vi "S4GUI.vi"() -> ()   [LabVIEW 2018] (continued)
                n1821 = call-dynamic "save config.vi"("error in (no error)"=w4317, "file config"="lastsaved.cfg", "Channel in"=w4322) -> ("error out"=w4274:errorcluster, "Channel out"=w4279:refnum<class "Channel.lvclass">)  [unwired: 7 in]
                n1822 = local read "Filter2"() -> (w4273:u8)
                n1823 = call-dynamic "Write Filter.vi"("error in (no error)"=w4274, "Filter"=w4273, "Channel in"=w4279) -> ("error out"=w4292:errorcluster, "Channel out"=w4278:refnum<class "Channel.lvclass">)  [unwired: 7 in]
                n1824 = call-dynamic "Read Interface.vi"("error in (no error)"=w4292, "Channel in"=w4278) -> ("error out"=w4289:errorcluster, "Interface.lvclass"=w4288:refnum<class "Interface.lvclass">, "Channel out"=w4277:refnum<class "Channel.lvclass">)  [unwired: 7 in]
                n1825 = call-dynamic "Write Suffix.vi"("error in (no error)"=w4289, "Suffix"=w4272, "Interface in"=w4288) -> ("error out"=w4280:errorcluster, "Interface out"=w4283:refnum<class "Interface.lvclass">)  [unwired: 7 in]
                n1826 = call-dynamic "Write ObsType.vi"("error in (no error)"=w4280, "ObsType"=w4271, "Interface in"=w4283) -> ("error out"=w4281:errorcluster, "Interface out"=w4284:refnum<class "Interface.lvclass">)  [unwired: 7 in]
                n1827 = call-dynamic "Write Object.vi"("error in (no error)"=w4281, "Object"=w4270, "Interface in"=w4284) -> ("error out"=w4282:errorcluster, "Interface out"=w4285:refnum<class "Interface.lvclass">)  [unwired: 7 in]
                n1828 = call-dynamic "Write Comments.vi"("error in (no error)"=w4282, "Comments"=w4269, "Interface in"=w4285) -> ("error out"=w4286:errorcluster, "Interface out"=w4287:refnum<class "Interface.lvclass">)  [unwired: 7 in]
                n1829 = call-dynamic "Write Observer.vi"("error in (no error)"=w4286, "Observer"=w4268, "Interface in"=w4287) -> ("error out"=w4291:errorcluster, "Interface out"=w4290:refnum<class "Interface.lvclass">)  [unwired: 7 in]
                n1830 = call-dynamic "Write Interface.vi"("error in (no error)"=w4291, "Interface.lvclass"=w4290, "Channel in"=w4277) -> ("error out"=w4275:errorcluster, "Channel out"=w4276:refnum<class "Channel.lvclass">)  [unwired: 7 in]
                n1831 = call-dynamic "Read State Machine.vi"("error in (no error)"=w4275, "Device in"=w4276) -> ("error out"=w4314:errorcluster, "State Machine.lvclass"=w4324:refnum<class "State Machine.lvclass">, "Device out"=w4323:refnum<class "Channel.lvclass">)  [unwired: 7 in]
                n1832 = call-dynamic "Write State.vi"("error in (no error)"=w4314, "State"=60, "State Machine in"=w4324) -> ("error out"=w4315:errorcluster, "State Machine out"=w4325:refnum<class "State Machine.lvclass">)  [unwired: 7 in]
                n1833 = call-dynamic "Write State Machine.vi"("error in (no error)"=w4315, "State Machine.lvclass"=w4325, "Device in"=w4323) -> ("error out"=w4327:errorcluster, "Device out"=w4326:refnum<class "Channel.lvclass">)  [unwired: 7 in]
                n1834 = call-dynamic "Write Channel.vi"("error in (no error)"=w4327, "Channel.lvclass"=w4326, "Acquisition in"=w4298) -> ("error out"=w4293:errorcluster, "Acquisition out"=w4294:refnum<class "Acquisition.lvclass">)  [unwired: 7 in]
              }
            }
            n1835 = case shown="True" w4124 {
              tunnel: [w4328 w4385] -> w4135
              tunnel: [w4329 w4384] -> w4136
              tunnel: w4126 -> [w4329 w4356]
              tunnel: w4125 -> [w4328 w4355]
              tunnel: w4108 -> [_ w4334]
              tunnel: w4107 -> [_ w4333]
              tunnel: w4106 -> [_ w4332]
              tunnel: w4105 -> [_ w4331]
              tunnel: w4104 -> [_ w4330]
              frame False {
              }
              frame True {
                # "nome do arquivo .cfg"
                # "seção no arquivo .cfg"
                # "open"
                n1836 = call-dynamic "Read Channel.vi"("error in (no error)"=w4355, "Acquisition in"=w4356) -> ("error out"=w4386:errorcluster, "Channel.lvclass"=w4387:refnum<class "Channel.lvclass">, "Acquisition out"=w4388:refnum<class "Acquisition.lvclass">)  [unwired: 7 in]
                n1837 = call-dynamic "Read Interface.vi"("error in (no error)"=w4386, "Channel in"=w4387) -> ("error out"=w4376:errorcluster, "Interface.lvclass"=w4375:refnum<class "Interface.lvclass">, "Channel out"=w4389:refnum<class "Channel.lvclass">)  [unwired: 7 in]
                n1838 = call-dynamic "Get CCD_Config.vi"("error in (no error)"=w4376, "Interface in"=w4375) -> ("error out"=w4379:errorcluster, "output cluster"=w4380:T24, "Interface out"=w4374:refnum<class "Interface.lvclass">)  [unwired: 7 in]
                n1839 = Bundle By Name(cluster=w4380, "SHUTTER_MODE"=u8 1) -> (w4378:T24)
                n1840 = call-dynamic "Set CCD_Config.vi"("error in (no error)"=w4379, "input cluster"=w4378, "Interface in"=w4374) -> ("error out"=w4381:errorcluster, "Interface out"=w4373:refnum<class "Interface.lvclass">)  [unwired: 7 in]
                n1841 = Flatten To String(anything=w4378, error in (no error)=w4381) -> (data string=w4383:string, error out=w4382:errorcluster)  [unwired: 2 in, 1 out]
                n1842 = call "Write flatted cluster.vi"("error in (no error)"=w4382, "flatted cluster"=w4383, "Interface in"=w4373) -> ("error out"=w4371:errorcluster, "Interface out"=w4372:refnum<class "Interface.lvclass">)  [unwired: 7 in]
                n1843 = call-dynamic "Write Interface.vi"("error in (no error)"=w4371, "Interface.lvclass"=w4372, "Channel in"=w4389) -> ("error out"=w4366:errorcluster, "Channel out"=w4365:refnum<class "Channel.lvclass">)  [unwired: 7 in]
                n1844 = call "Write section_name.vi"("error in (no error)"=w4366, "section_name"="CCD_ACS1", "Channel in"=w4365) -> ("error out"=w4367:errorcluster, "Channel out"=w4362:refnum<class "Channel.lvclass">)  [unwired: 7 in]
                n1845 = call-dynamic "save config.vi"("error in (no error)"=w4367, "file config"="lastsaved.cfg", "Channel in"=w4362) -> ("error out"=w4338:errorcluster, "Channel out"=w4337:refnum<class "Channel.lvclass">)  [unwired: 7 in]
                n1846 = local read "Filter1"() -> (w4339:u8)
                n1847 = call-dynamic "Write Filter.vi"("error in (no error)"=w4338, "Filter"=w4339, "Channel in"=w4337) -> ("error out"=w4354:errorcluster, "Channel out"=w4353:refnum<class "Channel.lvclass">)  [unwired: 7 in]
                n1848 = call-dynamic "Read Interface.vi"("error in (no error)"=w4354, "Channel in"=w4353) -> ("error out"=w4350:errorcluster, "Interface.lvclass"=w4349:refnum<class "Interface.lvclass">, "Channel out"=w4343:refnum<class "Channel.lvclass">)  [unwired: 7 in]
                n1849 = call-dynamic "Write Suffix.vi"("error in (no error)"=w4350, "Suffix"=w4334, "Interface in"=w4349) -> ("error out"=w4340:errorcluster, "Interface out"=w4344:refnum<class "Interface.lvclass">)  [unwired: 7 in]
                n1850 = call-dynamic "Write ObsType.vi"("error in (no error)"=w4340, "ObsType"=w4333, "Interface in"=w4344) -> ("error out"=w4341:errorcluster, "Interface out"=w4345:refnum<class "Interface.lvclass">)  [unwired: 7 in]
                n1851 = call-dynamic "Write Object.vi"("error in (no error)"=w4341, "Object"=w4332, "Interface in"=w4345) -> ("error out"=w4342:errorcluster, "Interface out"=w4346:refnum<class "Interface.lvclass">)  [unwired: 7 in]
                n1852 = call-dynamic "Write Comments.vi"("error in (no error)"=w4342, "Comments"=w4331, "Interface in"=w4346) -> ("error out"=w4347:errorcluster, "Interface out"=w4348:refnum<class "Interface.lvclass">)  [unwired: 7 in]
                n1853 = call-dynamic "Write Observer.vi"("error in (no error)"=w4347, "Observer"=w4330, "Interface in"=w4348) -> ("error out"=w4352:errorcluster, "Interface out"=w4351:refnum<class "Interface.lvclass">)  [unwired: 7 in]
                n1854 = call-dynamic "Write Interface.vi"("error in (no error)"=w4352, "Interface.lvclass"=w4351, "Channel in"=w4343) -> ("error out"=w4335:errorcluster, "Channel out"=w4336:refnum<class "Channel.lvclass">)  [unwired: 7 in]
                n1855 = call-dynamic "Read State Machine.vi"("error in (no error)"=w4335, "Device in"=w4336) -> ("error out"=w4370:errorcluster, "State Machine.lvclass"=w4360:refnum<class "State Machine.lvclass">, "Device out"=w4361:refnum<class "Channel.lvclass">)  [unwired: 7 in]
                n1856 = call-dynamic "Write State.vi"("error in (no error)"=w4370, "State"=60, "State Machine in"=w4360) -> ("error out"=w4369:errorcluster, "State Machine out"=w4359:refnum<class "State Machine.lvclass">)  [unwired: 7 in]
                n1857 = call-dynamic "Write State Machine.vi"("error in (no error)"=w4369, "State Machine.lvclass"=w4359, "Device in"=w4361) -> ("error out"=w4357:errorcluster, "Device out"=w4358:refnum<class "Channel.lvclass">)  [unwired: 7 in]
                n1858 = call-dynamic "Write Channel.vi"("error in (no error)"=w4357, "Channel.lvclass"=w4358, "Acquisition in"=w4388) -> ("error out"=w4385:errorcluster, "Acquisition out"=w4384:refnum<class "Acquisition.lvclass">)  [unwired: 7 in]
              }
            }
            n1859 = case shown="True" w4118 {
              tunnel: w4120 -> [w4205 w4234]
              tunnel: w4119 -> [w4204 w4233]
              tunnel: [w4205 w4232] -> w4132
              tunnel: [w4204 w4231] -> w4131
              tunnel: w4108 -> [_ w4210]
              tunnel: w4107 -> [_ w4209]
              tunnel: w4106 -> [_ w4208]
              tunnel: w4105 -> [_ w4207]
              tunnel: w4104 -> [_ w4206]
              frame False {
              }
              frame True {
                # "nome do arquivo .cfg"
                # "seção no arquivo .cfg"
                # "open"
                n1860 = call-dynamic "Read Channel.vi"("error in (no error)"=w4233, "Acquisition in"=w4234) -> ("error out"=w4238:errorcluster, "Channel.lvclass"=w4237:refnum<class "Channel.lvclass">, "Acquisition out"=w4236:refnum<class "Acquisition.lvclass">)  [unwired: 7 in]
                n1861 = call-dynamic "Read Interface.vi"("error in (no error)"=w4238, "Channel in"=w4237) -> ("error out"=w4246:errorcluster, "Interface.lvclass"=w4247:refnum<class "Interface.lvclass">, "Channel out"=w4235:refnum<class "Channel.lvclass">)  [unwired: 7 in]
                n1862 = call-dynamic "Get CCD_Config.vi"("error in (no error)"=w4246, "Interface in"=w4247) -> ("error out"=w4243:errorcluster, "output cluster"=w4242:T24, "Interface out"=w4248:refnum<class "Interface.lvclass">)  [unwired: 7 in]
                n1863 = Bundle By Name(cluster=w4242, "SHUTTER_MODE"=u8 1) -> (w4244:T24)
                n1864 = call-dynamic "Set CCD_Config.vi"("error in (no error)"=w4243, "input cluster"=w4244, "Interface in"=w4248) -> ("error out"=w4241:errorcluster, "Interface out"=w4249:refnum<class "Interface.lvclass">)  [unwired: 7 in]
                n1865 = Flatten To String(anything=w4244, error in (no error)=w4241) -> (data string=w4239:string, error out=w4240:errorcluster)  [unwired: 2 in, 1 out]
                n1866 = call "Write flatted cluster.vi"("error in (no error)"=w4240, "flatted cluster"=w4239, "Interface in"=w4249) -> ("error out"=w4251:errorcluster, "Interface out"=w4250:refnum<class "Interface.lvclass">)  [unwired: 7 in]
                n1867 = call-dynamic "Write Interface.vi"("error in (no error)"=w4251, "Interface.lvclass"=w4250, "Channel in"=w4235) -> ("error out"=w4256:errorcluster, "Channel out"=w4257:refnum<class "Channel.lvclass">)  [unwired: 7 in]
                n1868 = call "Write section_name.vi"("error in (no error)"=w4256, "section_name"="CCD_ACS3", "Channel in"=w4257) -> ("error out"=w4255:errorcluster, "Channel out"=w4260:refnum<class "Channel.lvclass">)  [unwired: 7 in]
                n1869 = call-dynamic "save config.vi"("error in (no error)"=w4255, "file config"="lastsaved.cfg", "Channel in"=w4260) -> ("error out"=w4212:errorcluster, "Channel out"=w4215:refnum<class "Channel.lvclass">)  [unwired: 7 in]
                n1870 = local read "Filter3"() -> (w4211:u8)
                n1871 = call-dynamic "Write Filter.vi"("error in (no error)"=w4212, "Filter"=w4211, "Channel in"=w4215) -> ("error out"=w4216:errorcluster, "Channel out"=w4229:refnum<class "Channel.lvclass">)  [unwired: 7 in]
                n1872 = call-dynamic "Read Interface.vi"("error in (no error)"=w4216, "Channel in"=w4229) -> ("error out"=w4219:errorcluster, "Interface.lvclass"=w4220:refnum<class "Interface.lvclass">, "Channel out"=w4230:refnum<class "Channel.lvclass">)  [unwired: 7 in]
                n1873 = call-dynamic "Write Suffix.vi"("error in (no error)"=w4219, "Suffix"=w4210, "Interface in"=w4220) -> ("error out"=w4228:errorcluster, "Interface out"=w4225:refnum<class "Interface.lvclass">)  [unwired: 7 in]
                n1874 = call-dynamic "Write ObsType.vi"("error in (no error)"=w4228, "ObsType"=w4209, "Interface in"=w4225) -> ("error out"=w4227:errorcluster, "Interface out"=w4224:refnum<class "Interface.lvclass">)  [unwired: 7 in]
                n1875 = call-dynamic "Write Object.vi"("error in (no error)"=w4227, "Object"=w4208, "Interface in"=w4224) -> ("error out"=w4226:errorcluster, "Interface out"=w4223:refnum<class "Interface.lvclass">)  [unwired: 7 in]
                n1876 = call-dynamic "Write Comments.vi"("error in (no error)"=w4226, "Comments"=w4207, "Interface in"=w4223) -> ("error out"=w4222:errorcluster, "Interface out"=w4221:refnum<class "Interface.lvclass">)  [unwired: 7 in]
                n1877 = call-dynamic "Write Observer.vi"("error in (no error)"=w4222, "Observer"=w4206, "Interface in"=w4221) -> ("error out"=w4217:errorcluster, "Interface out"=w4218:refnum<class "Interface.lvclass">)  [unwired: 7 in]
                n1878 = call-dynamic "Write Interface.vi"("error in (no error)"=w4217, "Interface.lvclass"=w4218, "Channel in"=w4230) -> ("error out"=w4213:errorcluster, "Channel out"=w4214:refnum<class "Channel.lvclass">)  [unwired: 7 in]
                n1879 = call-dynamic "Read State Machine.vi"("error in (no error)"=w4213, "Device in"=w4214) -> ("error out"=w4252:errorcluster, "State Machine.lvclass"=w4262:refnum<class "State Machine.lvclass">, "Device out"=w4261:refnum<class "Channel.lvclass">)  [unwired: 7 in]
                n1880 = call-dynamic "Write State.vi"("error in (no error)"=w4252, "State"=60, "State Machine in"=w4262) -> ("error out"=w4253:errorcluster, "State Machine out"=w4263:refnum<class "State Machine.lvclass">)  [unwired: 7 in]
                n1881 = call-dynamic "Write State Machine.vi"("error in (no error)"=w4253, "State Machine.lvclass"=w4263, "Device in"=w4261) -> ("error out"=w4265:errorcluster, "Device out"=w4264:refnum<class "Channel.lvclass">)  [unwired: 7 in]
                n1882 = call-dynamic "Write Channel.vi"("error in (no error)"=w4265, "Channel.lvclass"=w4264, "Acquisition in"=w4236) -> ("error out"=w4231:errorcluster, "Acquisition out"=w4232:refnum<class "Acquisition.lvclass">)  [unwired: 7 in]
              }
            }
            n1883 = case shown="True" w4115 {
              tunnel: w4117 -> [w4143 w4172]
              tunnel: w4116 -> [w4142 w4171]
              tunnel: [w4143 w4170] -> w4130
              tunnel: [w4142 w4169] -> w4129
              tunnel: w4108 -> [_ w4148]
              tunnel: w4107 -> [_ w4147]
              tunnel: w4106 -> [_ w4146]
              tunnel: w4105 -> [_ w4145]
              tunnel: w4104 -> [_ w4144]
              frame False {
              }
              frame True {
                # "nome do arquivo .cfg"
                # "seção no arquivo .cfg"
                # "open"
                n1884 = call-dynamic "Read Channel.vi"("error in (no error)"=w4171, "Acquisition in"=w4172) -> ("error out"=w4200:errorcluster, "Channel.lvclass"=w4201:refnum<class "Channel.lvclass">, "Acquisition out"=w4202:refnum<class "Acquisition.lvclass">)  [unwired: 7 in]
                n1885 = call-dynamic "Read Interface.vi"("error in (no error)"=w4200, "Channel in"=w4201) -> ("error out"=w4192:errorcluster, "Interface.lvclass"=w4191:refnum<class "Interface.lvclass">, "Channel out"=w4203:refnum<class "Channel.lvclass">)  [unwired: 7 in]
                n1886 = call-dynamic "Get CCD_Config.vi"("error in (no error)"=w4192, "Interface in"=w4191) -> ("error out"=w4195:errorcluster, "output cluster"=w4196:T24, "Interface out"=w4190:refnum<class "Interface.lvclass">)  [unwired: 7 in]
                n1887 = Bundle By Name(cluster=w4196, "SHUTTER_MODE"=u8 1) -> (w4194:T24)
                n1888 = call-dynamic "Set CCD_Config.vi"("error in (no error)"=w4195, "input cluster"=w4194, "Interface in"=w4190) -> ("error out"=w4197:errorcluster, "Interface out"=w4189:refnum<class "Interface.lvclass">)  [unwired: 7 in]
                n1889 = Flatten To String(anything=w4194, error in (no error)=w4197) -> (data string=w4199:string, error out=w4198:errorcluster)  [unwired: 2 in, 1 out]
                n1890 = call "Write flatted cluster.vi"("error in (no error)"=w4198, "flatted cluster"=w4199, "Interface in"=w4189) -> ("error out"=w4187:errorcluster, "Interface out"=w4188:refnum<class "Interface.lvclass">)  [unwired: 7 in]
                n1891 = call-dynamic "Write Interface.vi"("error in (no error)"=w4187, "Interface.lvclass"=w4188, "Channel in"=w4203) -> ("error out"=w4182:errorcluster, "Channel out"=w4181:refnum<class "Channel.lvclass">)  [unwired: 7 in]
                n1892 = call "Write section_name.vi"("error in (no error)"=w4182, "section_name"="CCD_ACS4", "Channel in"=w4181) -> ("error out"=w4183:errorcluster, "Channel out"=w4178:refnum<class "Channel.lvclass">)  [unwired: 7 in]
                n1893 = call-dynamic "save config.vi"("error in (no error)"=w4183, "file config"="lastsaved.cfg", "Channel in"=w4178) -> ("error out"=w4150:errorcluster, "Channel out"=w4155:refnum<class "Channel.lvclass">)  [unwired: 7 in]
                n1894 = local read "Filter4"() -> (w4149:u8)
                n1895 = call-dynamic "Write Filter.vi"("error in (no error)"=w4150, "Filter"=w4149, "Channel in"=w4155) -> ("error out"=w4168:errorcluster, "Channel out"=w4154:refnum<class "Channel.lvclass">)  [unwired: 7 in]
                n1896 = call-dynamic "Read Interface.vi"("error in (no error)"=w4168, "Channel in"=w4154) -> ("error out"=w4165:errorcluster, "Interface.lvclass"=w4164:refnum<class "Interface.lvclass">, "Channel out"=w4153:refnum<class "Channel.lvclass">)  [unwired: 7 in]
                n1897 = call-dynamic "Write Suffix.vi"("error in (no error)"=w4165, "Suffix"=w4148, "Interface in"=w4164) -> ("error out"=w4156:errorcluster, "Interface out"=w4159:refnum<class "Interface.lvclass">)  [unwired: 7 in]
                n1898 = call-dynamic "Write ObsType.vi"("error in (no error)"=w4156, "ObsType"=w4147, "Interface in"=w4159) -> ("error out"=w4157:errorcluster, "Interface out"=w4160:refnum<class "Interface.lvclass">)  [unwired: 7 in]
                n1899 = call-dynamic "Write Object.vi"("error in (no error)"=w4157, "Object"=w4146, "Interface in"=w4160) -> ("error out"=w4158:errorcluster, "Interface out"=w4161:refnum<class "Interface.lvclass">)  [unwired: 7 in]
                n1900 = call-dynamic "Write Comments.vi"("error in (no error)"=w4158, "Comments"=w4145, "Interface in"=w4161) -> ("error out"=w4162:errorcluster, "Interface out"=w4163:refnum<class "Interface.lvclass">)  [unwired: 7 in]
                n1901 = call-dynamic "Write Observer.vi"("error in (no error)"=w4162, "Observer"=w4144, "Interface in"=w4163) -> ("error out"=w4167:errorcluster, "Interface out"=w4166:refnum<class "Interface.lvclass">)  [unwired: 7 in]
                n1902 = call-dynamic "Write Interface.vi"("error in (no error)"=w4167, "Interface.lvclass"=w4166, "Channel in"=w4153) -> ("error out"=w4151:errorcluster, "Channel out"=w4152:refnum<class "Channel.lvclass">)  [unwired: 7 in]
                n1903 = call-dynamic "Read State Machine.vi"("error in (no error)"=w4151, "Device in"=w4152) -> ("error out"=w4186:errorcluster, "State Machine.lvclass"=w4176:refnum<class "State Machine.lvclass">, "Device out"=w4177:refnum<class "Channel.lvclass">)  [unwired: 7 in]
                n1904 = call-dynamic "Write State.vi"("error in (no error)"=w4186, "State"=60, "State Machine in"=w4176) -> ("error out"=w4185:errorcluster, "State Machine out"=w4175:refnum<class "State Machine.lvclass">)  [unwired: 7 in]
                n1905 = call-dynamic "Write State Machine.vi"("error in (no error)"=w4185, "State Machine.lvclass"=w4175, "Device in"=w4177) -> ("error out"=w4173:errorcluster, "Device out"=w4174:refnum<class "Channel.lvclass">)  [unwired: 7 in]
                n1906 = call-dynamic "Write Channel.vi"("error in (no error)"=w4173, "Channel.lvclass"=w4174, "Acquisition in"=w4202) -> ("error out"=w4169:errorcluster, "Acquisition out"=w4170:refnum<class "Acquisition.lvclass">)  [unwired: 7 in]
              }
            }
            n1907 = disable-structure shown="Enabled" {
              frame Disabled {
                # "open"
                n1908 = local read "Input Cluster"() -> (w4139:T5)
                n1909 = Unbundle By Name(w4139) -> ("Parameters"=w4140:T23)
                n1910 = Bundle By Name(cluster=w4140, "Shutter\nMode"=u16 1 ("Shutter\nMode")) -> (w4137:T23)
                n1911 = Bundle By Name(cluster=w4139, "Parameters"=w4137) -> (w4138:T5)
                n1912 = local write "Input Cluster"(w4138) -> ()
              }
              frame Enabled {
              }
            }
          }
        }
        n1913 = call-dynamic "Write AcquisitionA.vi"("error in (no error)"=w3698, "Acquisition.lvclass"=w3699, "S4ACS_GUI in"=w3700) -> ("error out"=w3688:errorcluster, "S4ACS_GUI out"=w3692:refnum<class "S4GUI.lvclass">)  [unwired: 7 in]
        n1914 = call "Write AcquisitionB.vi"("error in (no error)"=w3693, "Acquisition.lvclass"=w3694, "S4ACS_GUI in"=w3692) -> ("error out"=w3687:errorcluster, "S4ACS_GUI out"=w3691:refnum<class "S4GUI.lvclass">)  [unwired: 7 in]
        n1915 = call-dynamic "Write AcquisitionC.vi"("error in (no error)"=w3682, "Acquisition.lvclass"=w3683, "S4ACS_GUI in"=w3691) -> ("error out"=w3686:errorcluster, "S4ACS_GUI out"=w3690:refnum<class "S4GUI.lvclass">)  [unwired: 7 in]
        n1916 = call-dynamic "Write AcquisitionD.vi"("error in (no error)"=w3680, "Acquisition.lvclass"=w3681, "S4ACS_GUI in"=w3690) -> ("error out"=w3685:errorcluster, "S4ACS_GUI out"=w3689:refnum<class "S4GUI.lvclass">)  [unwired: 7 in]
        n1917 = Merge Errors(w3688, w3687, w3686, w3685) -> (w3684:errorcluster)
        n1918 = call "Write cfg file.vi"("error in (no error)"=w3684, "cfg file"="lastsaved.cfg", "S4ACS_GUI in"=w3689) -> ("error out"=w3696:errorcluster, "S4ACS_GUI out"=w3695:refnum<class "S4GUI.lvclass">)  [unwired: 7 in]
      }
      event "Object_sflat", "Object_dark", "Object_zero", "Object_dflat", "Object_focus", "Object_obj": Value Change {
        n1919 = event-data() -> ("NewVal"=w4390:string)  [unwired: 1 in, 5 out]
        n1920 = stacked-sequence {
          seq-local: [w4426 _ _ _] -> [_ w4484 _ _]
          seq-local: [w4425 _ _ _] -> [_ w4483 _ _]
          seq-local: [_ w4482 _ _] -> [_ _ w4527 _]
          seq-local: [_ w4481 _ _] -> [_ _ w4526 _]
          seq-local: [_ _ w4525 _] -> [_ _ _ w4570]
          seq-local: [_ _ w4524 _] -> [_ _ _ w4569]
          tunnel: w4397 -> [w4438 _ _ _]
          tunnel: w4398 -> [w4437 _ _ _]
          tunnel: [_ _ _ w4568] -> w4392
          tunnel: [_ _ _ w4567] -> w4391
          tunnel: w4396 -> [w4424 w4480 w4523 w4566]
          tunnel: w4395 -> [w4423 w4479 w4509 w4552]
          tunnel: w4393 -> [w4422 w4465 w4508 w4551]
          tunnel: w4390 -> [w4421 w4464 w4507 w4550]
          tunnel: w4394 -> [w4420 w4463 w4506 w4549]
          frame #0 {
            # "observer"
            # "comment"
            # "object"
            # "suffix"
            # "obsType"
            n1921 = call-dynamic "Read AcquisitionA.vi"("error in (no error)"=w4438, "S4ACS_GUI in"=w4437) -> ("error out"=w4436:errorcluster, "Acquisition.lvclass"=w4435:refnum<class "Acquisition.lvclass">, "S4ACS_GUI out"=w4430:refnum<class "S4GUI.lvclass">)  [unwired: 7 in]
            n1922 = call-dynamic "Read Channel.vi"("error in (no error)"=w4436, "Acquisition in"=w4435) -> ("error out"=w4400:errorcluster, "Channel.lvclass"=w4403:refnum<class "Channel.lvclass">, "Acquisition out"=w4429:refnum<class "Acquisition.lvclass">)  [unwired: 7 in]
            n1923 = local read "Filter1"() -> (w4401:u8)
            n1924 = call-dynamic "Write Filter.vi"("error in (no error)"=w4400, "Filter"=w4401, "Channel in"=w4403) -> ("error out"=w4399:errorcluster, "Channel out"=w4402:refnum<class "Channel.lvclass">)  [unwired: 7 in]
            n1925 = call-dynamic "Read Interface.vi"("error in (no error)"=w4399, "Channel in"=w4402) -> ("error out"=w4416:errorcluster, "Interface.lvclass"=w4417:refnum<class "Interface.lvclass">, "Channel out"=w4434:refnum<class "Channel.lvclass">)  [unwired: 7 in]
            n1926 = call-dynamic "Write Suffix.vi"("error in (no error)"=w4416, "Suffix"=w4424, "Interface in"=w4417) -> ("error out"=w4441:errorcluster, "Interface out"=w4433:refnum<class "Interface.lvclass">)  [unwired: 7 in]
            n1927 = call-dynamic "Write ObsType.vi"("error in (no error)"=w4441, "ObsType"=w4422, "Interface in"=w4433) -> ("error out"=w4440:errorcluster, "Interface out"=w4432:refnum<class "Interface.lvclass">)  [unwired: 7 in]
            n1928 = call-dynamic "Write Object.vi"("error in (no error)"=w4440, "Object"=w4421, "Interface in"=w4432) -> ("error out"=w4439:errorcluster, "Interface out"=w4431:refnum<class "Interface.lvclass">)  [unwired: 7 in]
            n1929 = call-dynamic "Write Comments.vi"("error in (no error)"=w4439, "Comments"=w4423, "Interface in"=w4431) -> ("error out"=w4419:errorcluster, "Interface out"=w4418:refnum<class "Interface.lvclass">)  [unwired: 7 in]
            n1930 = call-dynamic "Write Observer.vi"("error in (no error)"=w4419, "Observer"=w4420, "Interface in"=w4418) -> ("error out"=w4414:errorcluster, "Interface out"=w4415:refnum<class "Interface.lvclass">)  [unwired: 7 in]
            n1931 = call-dynamic "Write Interface.vi"("error in (no error)"=w4414, "Interface.lvclass"=w4415, "Channel in"=w4434) -> ("error out"=w4410:errorcluster, "Channel out"=w4413:refnum<class "Channel.lvclass">)  [unwired: 7 in]
            n1932 = call-dynamic "Read State Machine.vi"("error in (no error)"=w4410, "Device in"=w4413) -> ("error out"=w4409:errorcluster, "State Machine.lvclass"=w4407:refnum<class "State Machine.lvclass">, "Device out"=w4412:refnum<class "Channel.lvclass">)  [unwired: 7 in]
            n1933 = call "Next State.vi"("error in (no error)"=w4409, "New_State"=12, "State Machine in"=w4407) -> ("error out"=w4408:errorcluster, "State Machine out"=w4406:refnum<class "State Machine.lvclass">)  [unwired: 7 in]
            n1934 = call-dynamic "Write State Machine.vi"("error in (no error)"=w4408, "State Machine.lvclass"=w4406, "Device in"=w4412) -> ("error out"=w4405:errorcluster, "Device out"=w4411:refnum<class "Channel.lvclass">)  [unwired: 7 in]
            n1935 = call-dynamic "Write Channel.vi"("error in (no error)"=w4405, "Channel.lvclass"=w4411, "Acquisition in"=w4429) -> ("error out"=w4427:errorcluster, "Acquisition out"=w4428:refnum<class "Acquisition.lvclass">)  [unwired: 7 in]
            n1936 = call-dynamic "Write AcquisitionA.vi"("error in (no error)"=w4427, "Acquisition.lvclass"=w4428, "S4ACS_GUI in"=w4430) -> ("error out"=w4425:errorcluster, "S4ACS_GUI out"=w4426:refnum<class "S4GUI.lvclass">)  [unwired: 7 in]
          }
          frame #1 {
            # "object"
            # "suffix"
            # "obsType"
            n1937 = call "Read AcquisitionB.vi"("error in (no error)"=w4483, "S4ACS_GUI in"=w4484) -> ("error out"=w4469:errorcluster, "Acquisition.lvclass"=w4470:refnum<class "Acquisition.lvclass">, "S4ACS_GUI out"=w4475:refnum<class "S4GUI.lvclass">)  [unwired: 7 in]
            n1938 = call-dynamic "Read Channel.vi"("error in (no error)"=w4469, "Acquisition in"=w4470) -> ("error out"=w4443:errorcluster, "Channel.lvclass"=w4445:refnum<class "Channel.lvclass">, "Acquisition out"=w4476:refnum<class "Acquisition.lvclass">)  [unwired: 7 in]
            n1939 = local read "Filter2"() -> (w4446:u8)
            n1940 = call-dynamic "Write Filter.vi"("error in (no error)"=w4443, "Filter"=w4446, "Channel in"=w4445) -> ("error out"=w4442:errorcluster, "Channel out"=w4444:refnum<class "Channel.lvclass">)  [unwired: 7 in]
            n1941 = call-dynamic "Read Interface.vi"("error in (no error)"=w4442, "Channel in"=w4444) -> ("error out"=w4457:errorcluster, "Interface.lvclass"=w4458:refnum<class "Interface.lvclass">, "Channel out"=w4471:refnum<class "Channel.lvclass">)  [unwired: 7 in]
            n1942 = call-dynamic "Write Suffix.vi"("error in (no error)"=w4457, "Suffix"=w4480, "Interface in"=w4458) -> ("error out"=w4466:errorcluster, "Interface out"=w4472:refnum<class "Interface.lvclass">)  [unwired: 7 in]
            n1943 = call-dynamic "Write ObsType.vi"("error in (no error)"=w4466, "ObsType"=w4465, "Interface in"=w4472) -> ("error out"=w4467:errorcluster, "Interface out"=w4473:refnum<class "Interface.lvclass">)  [unwired: 7 in]
            n1944 = call-dynamic "Write Object.vi"("error in (no error)"=w4467, "Object"=w4464, "Interface in"=w4473) -> ("error out"=w4468:errorcluster, "Interface out"=w4474:refnum<class "Interface.lvclass">)  [unwired: 7 in]
            n1945 = call-dynamic "Write Comments.vi"("error in (no error)"=w4468, "Comments"=w4479, "Interface in"=w4474) -> ("error out"=w4460:errorcluster, "Interface out"=w4459:refnum<class "Interface.lvclass">)  [unwired: 7 in]
            n1946 = call-dynamic "Write Observer.vi"("error in (no error)"=w4460, "Observer"=w4463, "Interface in"=w4459) -> ("error out"=w4461:errorcluster, "Interface out"=w4462:refnum<class "Interface.lvclass">)  [unwired: 7 in]
            n1947 = call-dynamic "Write Interface.vi"("error in (no error)"=w4461, "Interface.lvclass"=w4462, "Channel in"=w4471) -> ("error out"=w4450:errorcluster, "Channel out"=w4451:refnum<class "Channel.lvclass">)  [unwired: 7 in]
            n1948 = call-dynamic "Read State Machine.vi"("error in (no error)"=w4450, "Device in"=w4451) -> ("error out"=w4456:errorcluster, "State Machine.lvclass"=w4454:refnum<class "State Machine.lvclass">, "Device out"=w4449:refnum<class "Channel.lvclass">)  [unwired: 7 in]
            n1949 = call "Next State.vi"("error in (no error)"=w4456, "New_State"=12, "State Machine in"=w4454) -> ("error out"=w4455:errorcluster, "State Machine out"=w4453:refnum<class "State Machine.lvclass">)  [unwired: 7 in]
            n1950 = call-dynamic "Write State Machine.vi"("error in (no error)"=w4455, "State Machine.lvclass"=w4453, "Device in"=w4449) -> ("error out"=w4447:errorcluster, "Device out"=w4448:refnum<class "Channel.lvclass">)  [unwired: 7 in]
            n1951 = call-dynamic "Write Channel.vi"("error in (no error)"=w4447, "Channel.lvclass"=w4448, "Acquisition in"=w4476) -> ("error out"=w4478:errorcluster, "Acquisition out"=w4477:refnum<class "Acquisition.lvclass">)  [unwired: 7 in]
            n1952 = call "Write AcquisitionB.vi"("error in (no error)"=w4478, "Acquisition.lvclass"=w4477, "S4ACS_GUI in"=w4475) -> ("error out"=w4481:errorcluster, "S4ACS_GUI out"=w4482:refnum<class "S4GUI.lvclass">)  [unwired: 7 in]
          }
          frame #2 {
            # "object"
            # "suffix"
            # "obsType"
            n1953 = call-dynamic "Read AcquisitionC.vi"("error in (no error)"=w4526, "S4ACS_GUI in"=w4527) -> ("error out"=w4519:errorcluster, "Acquisition.lvclass"=w4518:refnum<class "Acquisition.lvclass">, "S4ACS_GUI out"=w4513:refnum<class "S4GUI.lvclass">)  [unwired: 7 in]
            n1954 = call-dynamic "Read Channel.vi"("error in (no error)"=w4519, "Acquisition in"=w4518) -> ("error out"=w4486:errorcluster, "Channel.lvclass"=w4488:refnum<class "Channel.lvclass">, "Acquisition out"=w4512:refnum<class "Acquisition.lvclass">)  [unwired: 7 in]
            n1955 = local read "Filter3"() -> (w4489:u8)
            n1956 = call-dynamic "Write Filter.vi"("error in (no error)"=w4486, "Filter"=w4489, "Channel in"=w4488) -> ("error out"=w4485:errorcluster, "Channel out"=w4487:refnum<class "Channel.lvclass">)  [unwired: 7 in]
            n1957 = call-dynamic "Read Interface.vi"("error in (no error)"=w4485, "Channel in"=w4487) -> ("error out"=w4504:errorcluster, "Interface.lvclass"=w4505:refnum<class "Interface.lvclass">, "Channel out"=w4517:refnum<class "Channel.lvclass">)  [unwired: 7 in]
            n1958 = call-dynamic "Write Suffix.vi"("error in (no error)"=w4504, "Suffix"=w4523, "Interface in"=w4505) -> ("error out"=w4522:errorcluster, "Interface out"=w4516:refnum<class "Interface.lvclass">)  [unwired: 7 in]
            n1959 = call-dynamic "Write ObsType.vi"("error in (no error)"=w4522, "ObsType"=w4508, "Interface in"=w4516) -> ("error out"=w4521:errorcluster, "Interface out"=w4515:refnum<class "Interface.lvclass">)  [unwired: 7 in]
            n1960 = call-dynamic "Write Object.vi"("error in (no error)"=w4521, "Object"=w4507, "Interface in"=w4515) -> ("error out"=w4520:errorcluster, "Interface out"=w4514:refnum<class "Interface.lvclass">)  [unwired: 7 in]
            n1961 = call-dynamic "Write Comments.vi"("error in (no error)"=w4520, "Comments"=w4509, "Interface in"=w4514) -> ("error out"=w4501:errorcluster, "Interface out"=w4500:refnum<class "Interface.lvclass">)  [unwired: 7 in]
            n1962 = call-dynamic "Write Observer.vi"("error in (no error)"=w4501, "Observer"=w4506, "Interface in"=w4500) -> ("error out"=w4502:errorcluster, "Interface out"=w4503:refnum<class "Interface.lvclass">)  [unwired: 7 in]
            n1963 = call-dynamic "Write Interface.vi"("error in (no error)"=w4502, "Interface.lvclass"=w4503, "Channel in"=w4517) -> ("error out"=w4495:errorcluster, "Channel out"=w4496:refnum<class "Channel.lvclass">)  [unwired: 7 in]
            n1964 = call-dynamic "Read State Machine.vi"("error in (no error)"=w4495, "Device in"=w4496) -> ("error out"=w4499:errorcluster, "State Machine.lvclass"=w4492:refnum<class "State Machine.lvclass">, "Device out"=w4494:refnum<class "Channel.lvclass">)  [unwired: 7 in]
            n1965 = call "Next State.vi"("error in (no error)"=w4499, "New_State"=12, "State Machine in"=w4492) -> ("error out"=w4498:errorcluster, "State Machine out"=w4491:refnum<class "State Machine.lvclass">)  [unwired: 7 in]
            n1966 = call-dynamic "Write State Machine.vi"("error in (no error)"=w4498, "State Machine.lvclass"=w4491, "Device in"=w4494) -> ("error out"=w4490:errorcluster, "Device out"=w4493:refnum<class "Channel.lvclass">)  [unwired: 7 in]
            n1967 = call-dynamic "Write Channel.vi"("error in (no error)"=w4490, "Channel.lvclass"=w4493, "Acquisition in"=w4512) -> ("error out"=w4510:errorcluster, "Acquisition out"=w4511:refnum<class "Acquisition.lvclass">)  [unwired: 7 in]
            n1968 = call-dynamic "Write AcquisitionC.vi"("error in (no error)"=w4510, "Acquisition.lvclass"=w4511, "S4ACS_GUI in"=w4513) -> ("error out"=w4524:errorcluster, "S4ACS_GUI out"=w4525:refnum<class "S4GUI.lvclass">)  [unwired: 7 in]
          }
          frame #3 {
            # "object"
            # "suffix"
            # "obsType"
            n1969 = call-dynamic "Read AcquisitionD.vi"("error in (no error)"=w4569, "S4ACS_GUI in"=w4570) -> ("error out"=w4562:errorcluster, "Acquisition.lvclass"=w4561:refnum<class "Acquisition.lvclass">, "S4ACS_GUI out"=w4556:refnum<class "S4GUI.lvclass">)  [unwired: 7 in]
            n1970 = call-dynamic "Read Channel.vi"("error in (no error)"=w4562, "Acquisition in"=w4561) -> ("error out"=w4529:errorcluster, "Channel.lvclass"=w4531:refnum<class "Channel.lvclass">, "Acquisition out"=w4555:refnum<class "Acquisition.lvclass">)  [unwired: 7 in]
            n1971 = local read "Filter4"() -> (w4532:u8)
            n1972 = call-dynamic "Write Filter.vi"("error in (no error)"=w4529, "Filter"=w4532, "Channel in"=w4531) -> ("error out"=w4528:errorcluster, "Channel out"=w4530:refnum<class "Channel.lvclass">)  [unwired: 7 in]
            n1973 = call-dynamic "Read Interface.vi"("error in (no error)"=w4528, "Channel in"=w4530) -> ("error out"=w4547:errorcluster, "Interface.lvclass"=w4548:refnum<class "Interface.lvclass">, "Channel out"=w4560:refnum<class "Channel.lvclass">)  [unwired: 7 in]
            n1974 = call-dynamic "Write Suffix.vi"("error in (no error)"=w4547, "Suffix"=w4566, "Interface in"=w4548) -> ("error out"=w4565:errorcluster, "Interface out"=w4559:refnum<class "Interface.lvclass">)  [unwired: 7 in]
            n1975 = call-dynamic "Write ObsType.vi"("error in (no error)"=w4565, "ObsType"=w4551, "Interface in"=w4559) -> ("error out"=w4564:errorcluster, "Interface out"=w4558:refnum<class "Interface.lvclass">)  [unwired: 7 in]
            n1976 = call-dynamic "Write Object.vi"("error in (no error)"=w4564, "Object"=w4550, "Interface in"=w4558) -> ("error out"=w4563:errorcluster, "Interface out"=w4557:refnum<class "Interface.lvclass">)  [unwired: 7 in]
            n1977 = call-dynamic "Write Comments.vi"("error in (no error)"=w4563, "Comments"=w4552, "Interface in"=w4557) -> ("error out"=w4546:errorcluster, "Interface out"=w4545:refnum<class "Interface.lvclass">)  [unwired: 7 in]
            n1978 = call-dynamic "Write Observer.vi"("error in (no error)"=w4546, "Observer"=w4549, "Interface in"=w4545) -> ("error out"=w4541:errorcluster, "Interface out"=w4540:refnum<class "Interface.lvclass">)  [unwired: 7 in]
            n1979 = call-dynamic "Write Interface.vi"("error in (no error)"=w4541, "Interface.lvclass"=w4540, "Channel in"=w4560) -> ("error out"=w4536:errorcluster, "Channel out"=w4539:refnum<class "Channel.lvclass">)  [unwired: 7 in]
            n1980 = call-dynamic "Read State Machine.vi"("error in (no error)"=w4536, "Device in"=w4539) -> ("error out"=w4544:errorcluster, "State Machine.lvclass"=w4534:refnum<class "State Machine.lvclass">, "Device out"=w4538:refnum<class "Channel.lvclass">)  [unwired: 7 in]
            n1981 = call "Next State.vi"("error in (no error)"=w4544, "New_State"=12, "State Machine in"=w4534) -> ("error out"=w4543:errorcluster, "State Machine out"=w4533:refnum<class "State Machine.lvclass">)  [unwired: 7 in]
            n1982 = call-dynamic "Write State Machine.vi"("error in (no error)"=w4543, "State Machine.lvclass"=w4533, "Device in"=w4538) -> ("error out"=w4535:errorcluster, "Device out"=w4537:refnum<class "Channel.lvclass">)  [unwired: 7 in]
            n1983 = call-dynamic "Write Channel.vi"("error in (no error)"=w4535, "Channel.lvclass"=w4537, "Acquisition in"=w4555) -> ("error out"=w4553:errorcluster, "Acquisition out"=w4554:refnum<class "Acquisition.lvclass">)  [unwired: 7 in]
            n1984 = call-dynamic "Write AcquisitionD.vi"("error in (no error)"=w4553, "Acquisition.lvclass"=w4554, "S4ACS_GUI in"=w4556) -> ("error out"=w4567:errorcluster, "S4ACS_GUI out"=w4568:refnum<class "S4GUI.lvclass">)  [unwired: 7 in]
          }
        }
      }
      event "DFLAT Comments", "SFLAT Comments", "DARK Comments", "ZERO Comments", "FOCUS Comments", "OBJECT Comments": Value Change {
        n1985 = event-data() -> ("NewVal"=w4571:string)  [unwired: 1 in, 5 out]
        n1986 = stacked-sequence {
          seq-local: [w4607 _ _ _] -> [_ w4665 _ _]
          seq-local: [w4606 _ _ _] -> [_ w4664 _ _]
          seq-local: [_ w4663 _ _] -> [_ _ w4708 _]
          seq-local: [_ w4662 _ _] -> [_ _ w4707 _]
          seq-local: [_ _ w4706 _] -> [_ _ _ w4751]
          seq-local: [_ _ w4705 _] -> [_ _ _ w4750]
          tunnel: w4578 -> [w4619 _ _ _]
          tunnel: w4579 -> [w4618 _ _ _]
          tunnel: [_ _ _ w4749] -> w4573
          tunnel: [_ _ _ w4748] -> w4572
          tunnel: w4576 -> [w4605 w4661 w4704 w4747]
          tunnel: w4571 -> [w4604 w4660 w4690 w4733]
          tunnel: w4574 -> [w4603 w4646 w4689 w4732]
          tunnel: w4577 -> [w4602 w4645 w4688 w4731]
          tunnel: w4575 -> [w4601 w4644 w4687 w4730]
          frame #0 {
            # "observer"
            # "comment"
            # "object"
            # "suffix"
            # "obsType"
            n1987 = call-dynamic "Read AcquisitionA.vi"("error in (no error)"=w4619, "S4ACS_GUI in"=w4618) -> ("error out"=w4617:errorcluster, "Acquisition.lvclass"=w4616:refnum<class "Acquisition.lvclass">, "S4ACS_GUI out"=w4611:refnum<class "S4GUI.lvclass">)  [unwired: 7 in]
            n1988 = call-dynamic "Read Channel.vi"("error in (no error)"=w4617, "Acquisition in"=w4616) -> ("error out"=w4581:errorcluster, "Channel.lvclass"=w4584:refnum<class "Channel.lvclass">, "Acquisition out"=w4610:refnum<class "Acquisition.lvclass">)  [unwired: 7 in]
            n1989 = local read "Filter1"() -> (w4582:u8)
            n1990 = call-dynamic "Write Filter.vi"("error in (no error)"=w4581, "Filter"=w4582, "Channel in"=w4584) -> ("error out"=w4580:errorcluster, "Channel out"=w4583:refnum<class "Channel.lvclass">)  [unwired: 7 in]
            n1991 = call-dynamic "Read Interface.vi"("error in (no error)"=w4580, "Channel in"=w4583) -> ("error out"=w4597:errorcluster, "Interface.lvclass"=w4598:refnum<class "Interface.lvclass">, "Channel out"=w4615:refnum<class "Channel.lvclass">)  [unwired: 7 in]
            n1992 = call-dynamic "Write Suffix.vi"("error in (no error)"=w4597, "Suffix"=w4605, "Interface in"=w4598) -> ("error out"=w4622:errorcluster, "Interface out"=w4614:refnum<class "Interface.lvclass">)  [unwired: 7 in]
            n1993 = call-dynamic "Write ObsType.vi"("error in (no error)"=w4622, "ObsType"=w4603, "Interface in"=w4614) -> ("error out"=w4621:errorcluster, "Interface out"=w4613:refnum<class "Interface.lvclass">)  [unwired: 7 in]
            n1994 = call-dynamic "Write Object.vi"("error in (no error)"=w4621, "Object"=w4602, "Interface in"=w4613) -> ("error out"=w4620:errorcluster, "Interface out"=w4612:refnum<class "Interface.lvclass">)  [unwired: 7 in]
            n1995 = call-dynamic "Write Comments.vi"("error in (no error)"=w4620, "Comments"=w4604, "Interface in"=w4612) -> ("error out"=w4600:errorcluster, "Interface out"=w4599:refnum<class "Interface.lvclass">)  [unwired: 7 in]
            n1996 = call-dynamic "Write Observer.vi"("error in (no error)"=w4600, "Observer"=w4601, "Interface in"=w4599) -> ("error out"=w4595:errorcluster, "Interface out"=w4596:refnum<class "Interface.lvclass">)  [unwired: 7 in]
            n1997 = call-dynamic "Write Interface.vi"("error in (no error)"=w4595, "Interface.lvclass"=w4596, "Channel in"=w4615) -> ("error out"=w4591:errorcluster, "Channel out"=w4594:refnum<class "Channel.lvclass">)  [unwired: 7 in]
            n1998 = call-dynamic "Read State Machine.vi"("error in (no error)"=w4591, "Device in"=w4594) -> ("error out"=w4590:errorcluster, "State Machine.lvclass"=w4588:refnum<class "State Machine.lvclass">, "Device out"=w4593:refnum<class "Channel.lvclass">)  [unwired: 7 in]
            n1999 = call "Next State.vi"("error in (no error)"=w4590, "New_State"=12, "State Machine in"=w4588) -> ("error out"=w4589:errorcluster, "State Machine out"=w4587:refnum<class "State Machine.lvclass">)  [unwired: 7 in]
            n2000 = call-dynamic "Write State Machine.vi"("error in (no error)"=w4589, "State Machine.lvclass"=w4587, "Device in"=w4593) -> ("error out"=w4586:errorcluster, "Device out"=w4592:refnum<class "Channel.lvclass">)  [unwired: 7 in]
            n2001 = call-dynamic "Write Channel.vi"("error in (no error)"=w4586, "Channel.lvclass"=w4592, "Acquisition in"=w4610) -> ("error out"=w4608:errorcluster, "Acquisition out"=w4609:refnum<class "Acquisition.lvclass">)  [unwired: 7 in]
            n2002 = call-dynamic "Write AcquisitionA.vi"("error in (no error)"=w4608, "Acquisition.lvclass"=w4609, "S4ACS_GUI in"=w4611) -> ("error out"=w4606:errorcluster, "S4ACS_GUI out"=w4607:refnum<class "S4GUI.lvclass">)  [unwired: 7 in]
          }
          frame #1 {
            # "object"
            # "suffix"
            # "obsType"
            n2003 = call "Read AcquisitionB.vi"("error in (no error)"=w4664, "S4ACS_GUI in"=w4665) -> ("error out"=w4650:errorcluster, "Acquisition.lvclass"=w4651:refnum<class "Acquisition.lvclass">, "S4ACS_GUI out"=w4656:refnum<class "S4GUI.lvclass">)  [unwired: 7 in]
            n2004 = call-dynamic "Read Channel.vi"("error in (no error)"=w4650, "Acquisition in"=w4651) -> ("error out"=w4624:errorcluster, "Channel.lvclass"=w4626:refnum<class "Channel.lvclass">, "Acquisition out"=w4657:refnum<class "Acquisition.lvclass">)  [unwired: 7 in]
            n2005 = local read "Filter2"() -> (w4627:u8)
            n2006 = call-dynamic "Write Filter.vi"("error in (no error)"=w4624, "Filter"=w4627, "Channel in"=w4626) -> ("error out"=w4623:errorcluster, "Channel out"=w4625:refnum<class "Channel.lvclass">)  [unwired: 7 in]
            n2007 = call-dynamic "Read Interface.vi"("error in (no error)"=w4623, "Channel in"=w4625) -> ("error out"=w4638:errorcluster, "Interface.lvclass"=w4639:refnum<class "Interface.lvclass">, "Channel out"=w4652:refnum<class "Channel.lvclass">)  [unwired: 7 in]
            n2008 = call-dynamic "Write Suffix.vi"("error in (no error)"=w4638, "Suffix"=w4661, "Interface in"=w4639) -> ("error out"=w4647:errorcluster, "Interface out"=w4653:refnum<class "Interface.lvclass">)  [unwired: 7 in]
            n2009 = call-dynamic "Write ObsType.vi"("error in (no error)"=w4647, "ObsType"=w4646, "Interface in"=w4653) -> ("error out"=w4648:errorcluster, "Interface out"=w4654:refnum<class "Interface.lvclass">)  [unwired: 7 in]
            n2010 = call-dynamic "Write Object.vi"("error in (no error)"=w4648, "Object"=w4645, "Interface in"=w4654) -> ("error out"=w4649:errorcluster, "Interface out"=w4655:refnum<class "Interface.lvclass">)  [unwired: 7 in]
            n2011 = call-dynamic "Write Comments.vi"("error in (no error)"=w4649, "Comments"=w4660, "Interface in"=w4655) -> ("error out"=w4641:errorcluster, "Interface out"=w4640:refnum<class "Interface.lvclass">)  [unwired: 7 in]
            n2012 = call-dynamic "Write Observer.vi"("error in (no error)"=w4641, "Observer"=w4644, "Interface in"=w4640) -> ("error out"=w4642:errorcluster, "Interface out"=w4643:refnum<class "Interface.lvclass">)  [unwired: 7 in]
            n2013 = call-dynamic "Write Interface.vi"("error in (no error)"=w4642, "Interface.lvclass"=w4643, "Channel in"=w4652) -> ("error out"=w4631:errorcluster, "Channel out"=w4632:refnum<class "Channel.lvclass">)  [unwired: 7 in]
            n2014 = call-dynamic "Read State Machine.vi"("error in (no error)"=w4631, "Device in"=w4632) -> ("error out"=w4637:errorcluster, "State Machine.lvclass"=w4635:refnum<class "State Machine.lvclass">, "Device out"=w4630:refnum<class "Channel.lvclass">)  [unwired: 7 in]
            n2015 = call "Next State.vi"("error in (no error)"=w4637, "New_State"=12, "State Machine in"=w4635) -> ("error out"=w4636:errorcluster, "State Machine out"=w4634:refnum<class "State Machine.lvclass">)  [unwired: 7 in]
            n2016 = call-dynamic "Write State Machine.vi"("error in (no error)"=w4636, "State Machine.lvclass"=w4634, "Device in"=w4630) -> ("error out"=w4628:errorcluster, "Device out"=w4629:refnum<class "Channel.lvclass">)  [unwired: 7 in]
            n2017 = call-dynamic "Write Channel.vi"("error in (no error)"=w4628, "Channel.lvclass"=w4629, "Acquisition in"=w4657) -> ("error out"=w4659:errorcluster, "Acquisition out"=w4658:refnum<class "Acquisition.lvclass">)  [unwired: 7 in]
            n2018 = call "Write AcquisitionB.vi"("error in (no error)"=w4659, "Acquisition.lvclass"=w4658, "S4ACS_GUI in"=w4656) -> ("error out"=w4662:errorcluster, "S4ACS_GUI out"=w4663:refnum<class "S4GUI.lvclass">)  [unwired: 7 in]
          }
          frame #2 {
            # "object"
            # "suffix"
            # "obsType"
            n2019 = call-dynamic "Read AcquisitionC.vi"("error in (no error)"=w4707, "S4ACS_GUI in"=w4708) -> ("error out"=w4700:errorcluster, "Acquisition.lvclass"=w4699:refnum<class "Acquisition.lvclass">, "S4ACS_GUI out"=w4694:refnum<class "S4GUI.lvclass">)  [unwired: 7 in]
            n2020 = call-dynamic "Read Channel.vi"("error in (no error)"=w4700, "Acquisition in"=w4699) -> ("error out"=w4667:errorcluster, "Channel.lvclass"=w4669:refnum<class "Channel.lvclass">, "Acquisition out"=w4693:refnum<class "Acquisition.lvclass">)  [unwired: 7 in]
            n2021 = local read "Filter3"() -> (w4670:u8)
            n2022 = call-dynamic "Write Filter.vi"("error in (no error)"=w4667, "Filter"=w4670, "Channel in"=w4669) -> ("error out"=w4666:errorcluster, "Channel out"=w4668:refnum<class "Channel.lvclass">)  [unwired: 7 in]
            n2023 = call-dynamic "Read Interface.vi"("error in (no error)"=w4666, "Channel in"=w4668) -> ("error out"=w4685:errorcluster, "Interface.lvclass"=w4686:refnum<class "Interface.lvclass">, "Channel out"=w4698:refnum<class "Channel.lvclass">)  [unwired: 7 in]
            n2024 = call-dynamic "Write Suffix.vi"("error in (no error)"=w4685, "Suffix"=w4704, "Interface in"=w4686) -> ("error out"=w4703:errorcluster, "Interface out"=w4697:refnum<class "Interface.lvclass">)  [unwired: 7 in]
            n2025 = call-dynamic "Write ObsType.vi"("error in (no error)"=w4703, "ObsType"=w4689, "Interface in"=w4697) -> ("error out"=w4702:errorcluster, "Interface out"=w4696:refnum<class "Interface.lvclass">)  [unwired: 7 in]
            n2026 = call-dynamic "Write Object.vi"("error in (no error)"=w4702, "Object"=w4688, "Interface in"=w4696) -> ("error out"=w4701:errorcluster, "Interface out"=w4695:refnum<class "Interface.lvclass">)  [unwired: 7 in]
            n2027 = call-dynamic "Write Comments.vi"("error in (no error)"=w4701, "Comments"=w4690, "Interface in"=w4695) -> ("error out"=w4682:errorcluster, "Interface out"=w4681:refnum<class "Interface.lvclass">)  [unwired: 7 in]
            n2028 = call-dynamic "Write Observer.vi"("error in (no error)"=w4682, "Observer"=w4687, "Interface in"=w4681) -> ("error out"=w4683:errorcluster, "Interface out"=w4684:refnum<class "Interface.lvclass">)  [unwired: 7 in]
            n2029 = call-dynamic "Write Interface.vi"("error in (no error)"=w4683, "Interface.lvclass"=w4684, "Channel in"=w4698) -> ("error out"=w4676:errorcluster, "Channel out"=w4677:refnum<class "Channel.lvclass">)  [unwired: 7 in]
            n2030 = call-dynamic "Read State Machine.vi"("error in (no error)"=w4676, "Device in"=w4677) -> ("error out"=w4680:errorcluster, "State Machine.lvclass"=w4673:refnum<class "State Machine.lvclass">, "Device out"=w4675:refnum<class "Channel.lvclass">)  [unwired: 7 in]
            n2031 = call "Next State.vi"("error in (no error)"=w4680, "New_State"=12, "State Machine in"=w4673) -> ("error out"=w4679:errorcluster, "State Machine out"=w4672:refnum<class "State Machine.lvclass">)  [unwired: 7 in]
            n2032 = call-dynamic "Write State Machine.vi"("error in (no error)"=w4679, "State Machine.lvclass"=w4672, "Device in"=w4675) -> ("error out"=w4671:errorcluster, "Device out"=w4674:refnum<class "Channel.lvclass">)  [unwired: 7 in]
            n2033 = call-dynamic "Write Channel.vi"("error in (no error)"=w4671, "Channel.lvclass"=w4674, "Acquisition in"=w4693) -> ("error out"=w4691:errorcluster, "Acquisition out"=w4692:refnum<class "Acquisition.lvclass">)  [unwired: 7 in]
            n2034 = call-dynamic "Write AcquisitionC.vi"("error in (no error)"=w4691, "Acquisition.lvclass"=w4692, "S4ACS_GUI in"=w4694) -> ("error out"=w4705:errorcluster, "S4ACS_GUI out"=w4706:refnum<class "S4GUI.lvclass">)  [unwired: 7 in]
          }
          frame #3 {
            # "object"
            # "suffix"
            # "obsType"
            n2035 = call-dynamic "Read AcquisitionD.vi"("error in (no error)"=w4750, "S4ACS_GUI in"=w4751) -> ("error out"=w4743:errorcluster, "Acquisition.lvclass"=w4742:refnum<class "Acquisition.lvclass">, "S4ACS_GUI out"=w4737:refnum<class "S4GUI.lvclass">)  [unwired: 7 in]
            n2036 = call-dynamic "Read Channel.vi"("error in (no error)"=w4743, "Acquisition in"=w4742) -> ("error out"=w4710:errorcluster, "Channel.lvclass"=w4712:refnum<class "Channel.lvclass">, "Acquisition out"=w4736:refnum<class "Acquisition.lvclass">)  [unwired: 7 in]
            n2037 = local read "Filter4"() -> (w4713:u8)
            n2038 = call-dynamic "Write Filter.vi"("error in (no error)"=w4710, "Filter"=w4713, "Channel in"=w4712) -> ("error out"=w4709:errorcluster, "Channel out"=w4711:refnum<class "Channel.lvclass">)  [unwired: 7 in]
            n2039 = call-dynamic "Read Interface.vi"("error in (no error)"=w4709, "Channel in"=w4711) -> ("error out"=w4728:errorcluster, "Interface.lvclass"=w4729:refnum<class "Interface.lvclass">, "Channel out"=w4741:refnum<class "Channel.lvclass">)  [unwired: 7 in]
